vi "Clear Slot.vi"(8 "error in":errorcluster, 11 "slot ref in":T1 format="%.0x") -> (0 "error out":errorcluster, 3 "slot ref out":T1 format="%.0x")   [LabVIEW 2020, in "Scan Engine Scripting.lvlib"]
doc: "Removes the existing module from the slot. The slot is left with an empty module."
uses:
  Scan Engine Scripting.lvlib
  <vilib>/NI VeriStand/Custom Device API/Custom Device Item Ref.ctl
  Modules.lvlibp/RSI Module/Module Models.ctl
  Modules.lvlibp/RSI Module/RSI Module.lvclass
  Custom Device Source/Modules.lvlibp
  <vilib>/NI VeriStand/Custom Device API/Custom Device API.lvlib
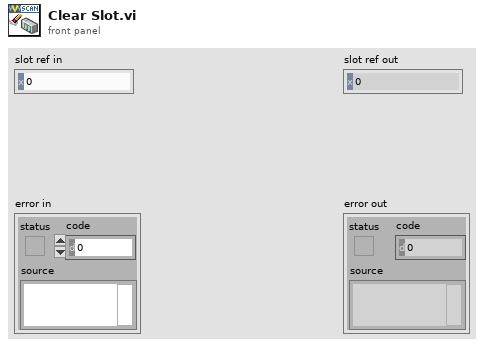
[diagram p1: front panel]
types:
  T1 = typedef "Custom Device API.lvlib/Custom Device Item Ref.ctl" = u64
  T2 = typedef "Modules.lvlibp/RSI Module.lvclass/Module Models.ctl" = enum16{"Empty", "NI 9201", "NI 9203", "NI 9205", "NI 9206", "NI 9207", "NI 9208", "NI 9209", "NI 9210", "NI 9211", "NI 9212", "NI 9213", "NI 9214", "NI 9215", "NI 9216", "NI 9217", "NI 9219", "NI 9220", "NI 9221", "NI 9222", "NI 9223", "NI 9224", "NI 9225", "NI 9226", "NI 9227", "NI 9228", "NI 9229", "NI 9233", "NI 9234", "NI 9235", "NI 9236", "NI 9237", "NI 9239", "NI 9242", "NI 9244", "NI 9253", "NI 9263", "NI 9264", "NI 9265", "NI 9266", "NI 9269", "NI 9344", "NI 9350", "NI 9375", "NI 9401", "NI 9402", "NI 9403", "NI 9411", "NI 9421", "NI 9422", "NI 9423", "NI 9425", "NI 9426", "NI 9435", "NI 9436", "NI 9437", "NI 9472", "NI 9474", "NI 9475", "NI 9476", "NI 9477", "NI 9478", "NI 9481", "NI 9482", "NI 9485"}
  T3 = typedef "Modules.lvlibp/Custom Device API.lvlib/Custom Device Item Ref.ctl" = u64
  T4 = typedef "Modules.lvlibp/RSI Module.lvclass/Slot Settings.ctl" = cluster{"Slot":u32, "EtherCAT?":bool}
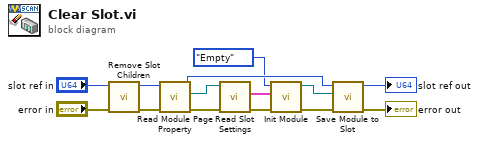
[diagram p0: block diagram]
diagram:
  n1 = call "Remove Slot Children.vi"("error in"="error in", "slot ref in"="slot ref in") -> ("error out"=w5:errorcluster, "slot ref out"=w3:T1)  [unwired: 8 in]
  n2 = call "Read Module Page Property.vi"("error in (no error)"=w5, "Node Ptr In"=w3) -> ("error out"=w14:errorcluster, "RSI Module"=w13:refnum<class "RSI Module.lvclass">, "Node Ptr Out"=w12:T3)  [unwired: 7 in]
  n3 = call "Read Slot Settings.vi"("error in (no error)"=w14, "RSI Module in"=w13) -> ("error out"=w11:errorcluster, "Slot Settings"=w10:T4)  [unwired: 7 in, 1 out]
  n4 = call "Init Module.vi"("error in (no error)"=w11, "Slot Settings"=w10, "Module Model"=Module_Models."Empty") -> ("error out"=w8:errorcluster, "RSI Module out"=w9:refnum<class "RSI Module.lvclass">)  [unwired: 7 in]
  n5 = call "Save Module to Slot.vi"("error in"=w8, "RSI module in"=w9, "slot ref in"=w12) -> ("error out"=→"error out":errorcluster, "slot ref out"=→"slot ref out":T3)  [unwired: 6 in, 1 out]
